vi "TD_Close_Connection.vi"(8 "error in (no error)":errorcluster, 11 "TekDrive Session":T1) -> (0 "error out":errorcluster)   [LabVIEW 2018]
uses:
  Controls/TekDriveSession.ctl
  <vilib>/httpClient/ClientHandle.ctl
  <vilib>/httpClient/LabVIEWHTTPClient.lvlib
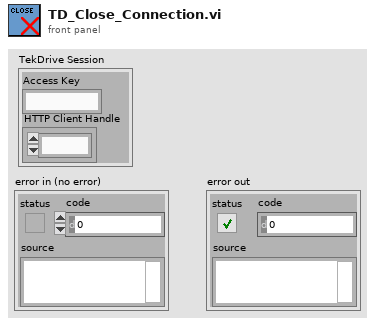
[diagram p1: front panel]
types:
  T1 = typedef "TekDriveSession.ctl" = cluster{"Access Key":string, "HTTP Client Handle":T2}
  T2 = typedef "LabVIEWHTTPClient.lvlib/ClientHandle.ctl" = refnum<k1>
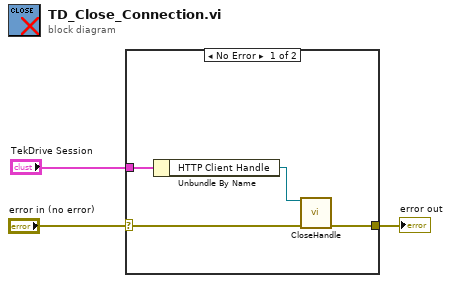
[diagram p0: block diagram]
diagram:
  n1 = case shown="No Error" "error in (no error)" {
    selector: "error in (no error)" -> [w7 w8]
    tunnel: "TekDrive Session" -> [w6 _]
    tunnel: [w4 w8] -> w1
    frame No Error {
      n2 = Unbundle By Name(w6) -> ("HTTP Client Handle"=w5:T2)
      n3 = call <vilib>:"CloseHandle.vi"("client handle"=w5, "error in (no error)"=w7) -> ("error out"=w4:errorcluster)  [unwired: 13 in]
    }
    frame Error {
    }
  }
  "error out" <- w1
